vi "Check tote in intake.vi"() -> (0 "Either":bool, 1 "Right":bool, 2 "Left":bool, 3 "Both":bool)   [LabVIEW 2014]
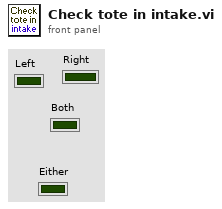
[diagram p1: front panel]
types:
  T1 = typedef "WPI_SwitchDevRef.ctl" = cluster{"DevStatus":errorcluster, "DIO Channel":T2, "Controller":T3, "CntIndex":T4, "Normally Closed":bool}
  T2 = typedef "FPGA_DIOChannel.ctl" = enum8{"DIO 0", "DIO 1", "DIO 2", "DIO 3", "DIO 4", "DIO 5", "DIO 6", "DIO 7", "DIO 8", "DIO 9", "DIO MXP 0", "DIO MXP 1", "DIO MXP 2", "DIO MXP 3", "DIO MXP 4", "DIO MXP 5", "DIO MXP 6", "DIO MXP 7", "DIO MXP 8", "DIO MXP 9", "DIO MXP 10", "DIO MXP 11", "DIO MXP 12", "DIO MXP 13", "DIO MXP 14", "DIO MXP 15", "Invalid"}
  T3 = typedef "FPGA_TypedefDigitalModule.ctl" = enum16{"Controller 1"}
  T4 = typedef "FPGA_CounterCtrSystemIndex.ctl" = enum8{"Ctr 0", "Ctr 1", "Ctr 2", "Ctr 3", "Ctr 4", "Ctr 5", "Ctr 6", "Ctr 7", "Invalid"}
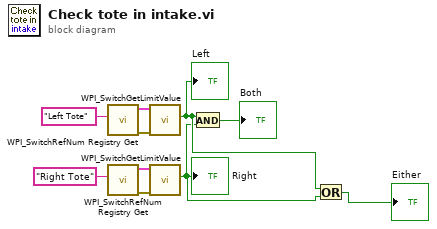
[diagram p0: block diagram]
diagram:
  n1 = call <vilib>:"WPI_SwitchRefNum Registry Get.vi"("refnum name"="Left Tote") -> ("error out"=w10:errorcluster, "SwitchDevRef"=w9:T1)  [unwired: 9 in]
  n2 = call <vilib>:"WPI_SwitchRefNum Registry Get.vi"("refnum name"="Right Tote") -> ("error out"=w5:errorcluster, "SwitchDevRef"=w6:T1)  [unwired: 9 in]
  n3 = call <vilib>:"WPI_SwitchGetLimitValue.vi"("error in (no error)"=w10, "SwitchDevRef"=w9) -> ("Switch Pressed"=w2:bool)  [unwired: 7 in, 2 out]
  "Left" <- w2
  n4 = call <vilib>:"WPI_SwitchGetLimitValue.vi"("error in (no error)"=w5, "SwitchDevRef"=w6) -> ("Switch Pressed"=w1:bool)  [unwired: 7 in, 2 out]
  "Right" <- w1
  n5 = And(x=w2, y=w1) -> (x .and. y?=→"Both":bool)
  n6 = Or(x=w2, y=w1) -> (x .or. y?=→"Either":bool)
